vi "Variant to Class.vi"(8 "error in (no error)":errorcluster, 10 "Data in":variant, 11 "LabVIEW Build Node in":refnum<class "LabVIEW Build Node.lvclass">) -> (0 "error out":errorcluster, 2 "Data Out":variant, 3 "LabVIEW Build Node out":refnum<class "LabVIEW Build Node.lvclass">)   [LabVIEW 2014, in "LabVIEW Build Node.lvclass"]
uses:
  LabVIEW Build Node.lvclass
  Shared/Controls/LabVIEW Build - STYP.ctl
  LabVIEW Build Node.lvclass/LabVIEW Build Node.ctl
  Classes/Build Job/Build Job.lvclass
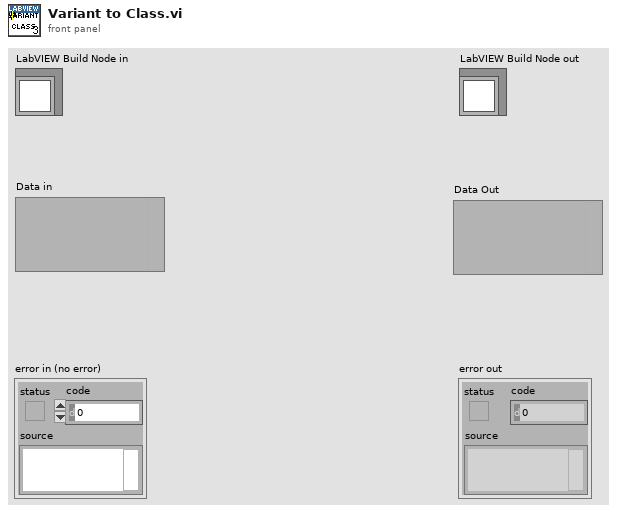
[diagram p1: front panel]
types:
  T1 = typedef "LabVIEW Build - STYP.ctl" = cluster{"Executor_Number":string, "Workspace_Path":string, "Build_Spec":string, "Target":string, "Project_Path":string, "Auto_Version_Increment":bool}
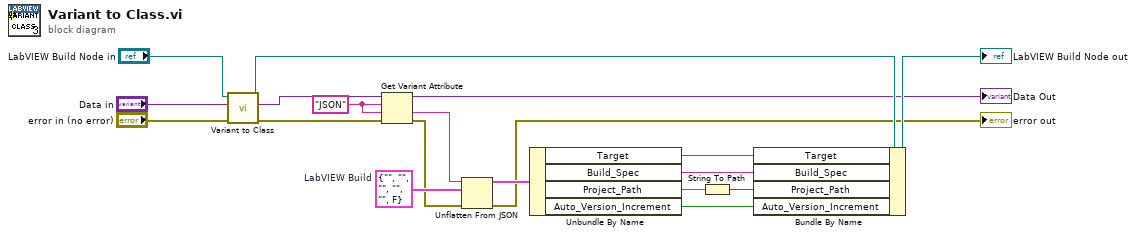
[diagram p0: block diagram]
diagram:
  w12 = T1 {"Executor_Number"="", "Workspace_Path"="", "Build_Spec"="", "Target"="", "Project_Path"="", "Auto_Version_Increment"=FALSE}  # LabVIEW Build
  w15 = "JSON" ("name")
  n1 = call-parent "Variant to Class.vi"("error in (no error)"="error in (no error)", "Data in"="Data in", "Build Job in"="LabVIEW Build Node in") -> ("error out"=w5:errorcluster, "Data Out"=w16:variant, "Build Job out"=w14:refnum<class "LabVIEW Build Node.lvclass">)  [unwired: 6 in]
  n2 = Get Variant Attribute(Variant=w16, name=w15, default value (empty Variant)=w15, error in=w5) -> (duplicate Variant=→"Data Out":variant, value=w13:string, error out=w4:errorcluster)  [unwired: 1 out]
  n3 = Unflatten From JSON(JSON string=w13, type and defaults=w12, error in (no error)=w4) -> (value=w10:T1, error out=→"error out":errorcluster)  [unwired: 4 in]
  n4 = Unbundle By Name(w10) -> ("Target"=w1:string, "Build_Spec"=w9:string, "Project_Path"=w8:string, "Auto_Version_Increment"=w7:bool)
  n5 = String To Path(string=w8) -> (path=w2:path)
  n6 = Bundle By Name(cluster=w14, "Target"=w1, "Build_Spec"=w9, "Project_Path"=w2, "Auto_Version_Increment"=w7) -> (→"LabVIEW Build Node out":refnum<class "LabVIEW Build Node.lvclass">)
